vi "Test Pdash Style.vi"() -> ()   [LabVIEW 2024]
uses:
  Control 1.ctl
  <vilib>/National Instruments/Tree Map/API/List Roots.vi
  <vilib>/National Instruments/Tree Map/Utility/Into Tree Control Items.vi
  <vilib>/National Instruments/Tree Map/Tree Map.lvlib
panel:
  in  "Numeric 3":dbl
  out "Tank 2":dbl(slide) scale=0.0..10.0
  in  "String Control":string
  in  "String 3":string
  in  "Button":bool
  in  "String":string="test text"
  in  "Tree Control":string(tree)
  out "Numeric 2":dbl
  in  "Numeric":dbl
  in  "Listbox":i32(listbox)
  in  "Results Listbox":T1
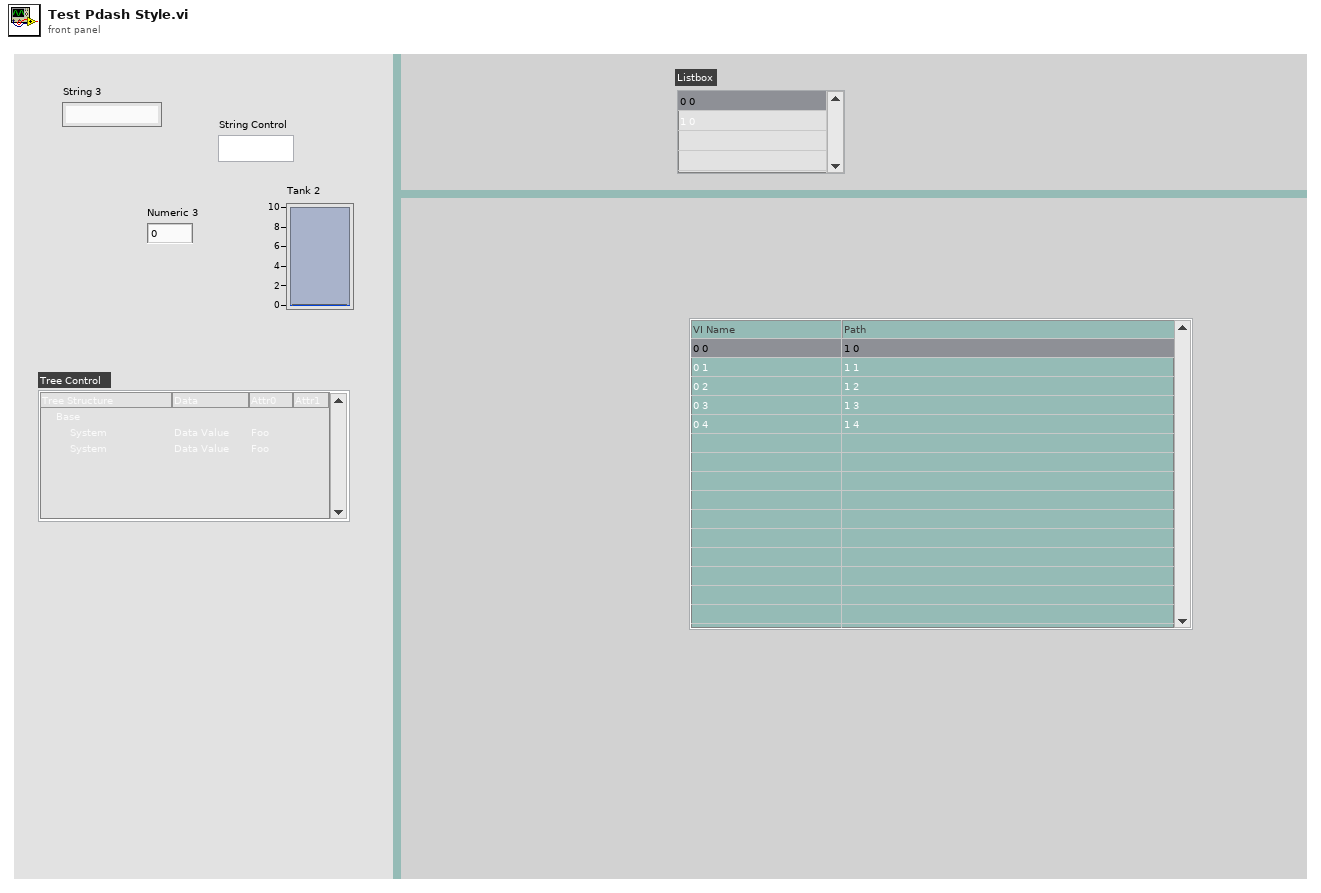
[diagram p1: front panel]
types:
  T1 = typedef "Control 1.ctl" = i32
  T2 = typedef "Tree Map.lvlib/Tree Map Data.ctl" = map{string, cluster{"Child Paths Set":set{string}, "Name":string, "Data":string, "Attributes":map{string, string}}}
  T3 = cluster{"Left Cell String":string, "Child Text":string[], "Child Tag":string, "Item Indent":i32, "Child Only?":bool, "Glyph Index":i32}[]
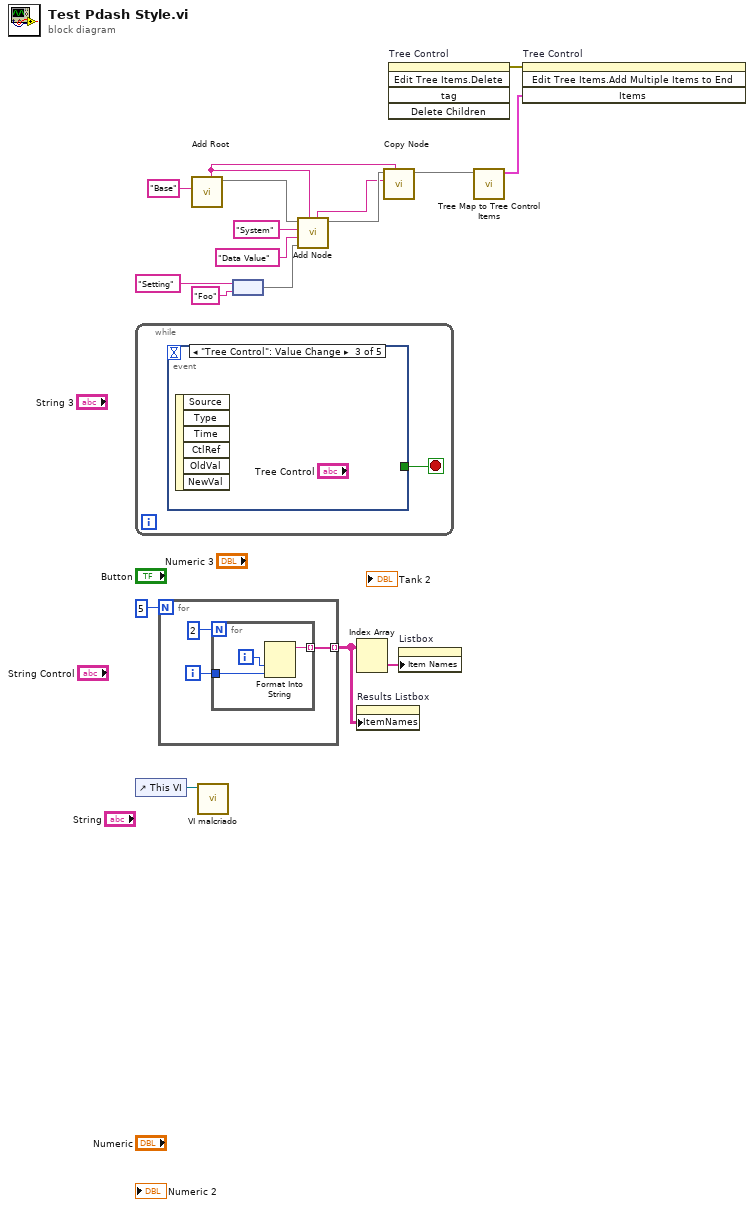
[diagram p0: block diagram]
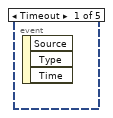
[diagram p2: hidden frame]
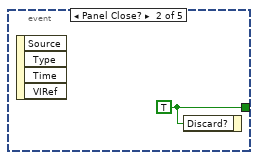
[diagram p3: hidden frame]
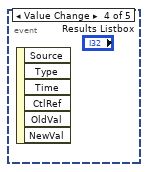
[diagram p4: hidden frame]
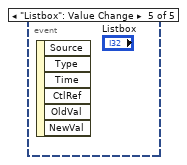
[diagram p5: hidden frame]
diagram:
  n1 = while {
    stop <- w18 stop-if-true
    n2 = event shown="[2] \"Tree Control\": Value Change" {
      selector: _ -> [_ _ _ _ _]
      dyn-events: _ -> [_ _ _ _ _]
      timeout: _ -> [_ _ _ _ _]
      tunnel: [_ w19 _ _ _] -> w18
      event Timeout {
        n3 = event-data() -> ()  [unwired: 1 in, 3 out]
      }
      event Panel Close? {
        w19 = TRUE ("Discard?")
        n4 = event-data() -> ()  [unwired: 1 in, 4 out]
        n5 = event-data("Discard?"=w19) -> ()  [unwired: 1 in, 1 out]
      }
      event "Tree Control": Value Change {
        n6 = event-data() -> ()  [unwired: 1 in, 6 out]
      }
      event Value Change {
        n7 = event-data() -> ()  [unwired: 1 in, 6 out]
      }
      event "Listbox": Value Change {
        n8 = event-data() -> ()  [unwired: 1 in, 6 out]
      }
    }
  }
  n9 = control-ref of="This VI"() -> (w1:refnum<vi>)
  n10 = for {
    N: 5 -> [_]
    tunnel: [w21] -> w3 mode=indexing
    i -> [w22]
    n11 = for {
      N: 2 -> [_]
      tunnel: w22 -> [w24]
      tunnel: [w23] -> w21 mode=indexing
      i -> [w25]
      n12 = Format Into String(w25, w24) -> (resulting string=w23:string)  [unwired: 3 in, 1 out]
    }
  }
  n13 = call <vilib>:"Add Root.vi"("New Root Name"="Base") -> ("Tree Map Out"=w15:T2, "Root Path"=w7:string)  [unwired: 9 in]
  n14 = call "VI malcriado.vi"("This VI"=w1) -> ()  [unwired: 11 in]
  n15 = node("Setting" ("New Root Name"), "Foo" ("New Root Name")) -> (w12:map{string, string})
  n16 = call <vilib>:"Add Node.vi"("Parent Path"=w7, "Attributes"=w12, "Data"="Data Value" ("New Root Name"), "New Node Name"="System" ("New Root Name"), "Tree Map In"=w15) -> ("Tree Map Out"=w6:T2, "New Node Path"=w5:string)  [unwired: 4 in, 1 out]
  n17 = Index Array(array=w3) -> (element=w2:string[])  [unwired: 2 in]
  n18 = property on="Results Listbox" class="MCListbox (strict)"("ItemNames"=w3) -> ()  [unwired: 2 in, 2 out]
  n19 = call <vilib>:"Copy Node.vi"("New Parent Path in Target"=w7, "Node Path in Source"=w5, "Target Tree Map In"=w6) -> ("Target Tree Map Out"=w8:T2)  [unwired: 6 in, 2 out]
  n20 = invoke on="Tree Control" class="Tree (strict)" method="Edit Tree Items.Delete"() -> (error out=w17:errorcluster)  [unwired: 5 in, 4 out]
  n21 = property on="Listbox" class="LstBox (strict)"("Item Names"=w2) -> ()  [unwired: 2 in, 2 out]
  n22 = call <vilib>:"Tree Map to Tree Control Items.vi"("Tree Map In"=w8) -> ("Tree Control Items"=w9:T3)  [unwired: 10 in]
  n23 = invoke on="Tree Control" class="Tree (strict)" method="Edit Tree Items.Add Multiple Items to End"(error in=w17, "Items"=w9) -> ()  [unwired: 2 in, 4 out]
